vi "RSToutput.vi"(6 "RST Motor Constants":T1={"Pitch Gain (2*pi/enc)"=1.0, "Output Sign"=[1.0, -1.0, 1.0], "Phase Offset (rad)"=0.0, "Saturation"=32000.0}, 9 "Encoder Position":dbl, 11 "Command":dbl) -> (1 "Coerced?":bool, 3 "Control":dbl[](array[numeric]))   [LabVIEW 2010, in "kevLib2010.lvlib"]
uses:
  kevLib2010.lvlib
  RSTtypeDef.ctl
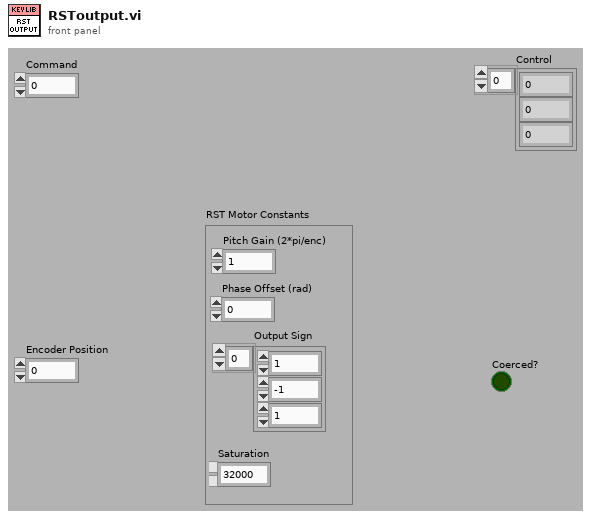
[diagram p1: front panel]
types:
  T1 = typedef "kevLib2010.lvlib/RSTtypeDef.ctl" = cluster{"Pitch Gain (2*pi/enc)":dbl, "Output Sign":dbl[], "Phase Offset (rad)":dbl, "Saturation":dbl}
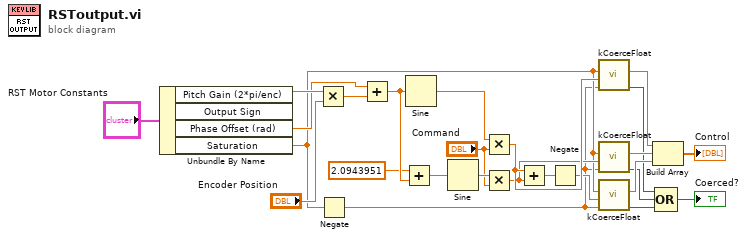
[diagram p0: block diagram]
diagram:
  n1 = Unbundle By Name("RST Motor Constants") -> ("Pitch Gain (2*pi/enc)"=w23:dbl, "Phase Offset (rad)"=w21:dbl, "Saturation"=w5:dbl)  [unwired: 1 out]
  n2 = Multiply(x=w23, y="Encoder Position") -> (x*y=w22:dbl)
  n3 = Negate(x=w5) -> (-x=w4:dbl)
  n4 = Add(x=w21, y=w22) -> (x+y=w3:dbl)
  n5 = Add(x=2.0943951, y=w3) -> (x+y=w2:dbl)
  n6 = Sine(x=w3) -> (sin(x)=w20:dbl)
  n7 = Sine(x=w2) -> (sin(x)=w19:dbl)
  n8 = Multiply(x=w20, y="Command") -> (x*y=w16:dbl)
  n9 = Multiply(x=w19, y="Command") -> (x*y=w14:dbl)
  n10 = Add(x=w16, y=w14) -> (x+y=w17:dbl)
  n11 = Negate(x=w17) -> (-x=w15:dbl)
  n12 = call "kCoerceFloat.vi"("lower"=w4, "input"=w16, "upper"=w5) -> ("coerced?"=w10:bool, "output"=w13:dbl)  [unwired: 7 in]
  n13 = call "kCoerceFloat.vi"("lower"=w4, "input"=w14, "upper"=w5) -> ("coerced?"=w9:bool, "output"=w12:dbl)  [unwired: 7 in]
  n14 = call "kCoerceFloat.vi"("lower"=w4, "input"=w15, "upper"=w5) -> ("coerced?"=w8:bool, "output"=w11:dbl)  [unwired: 7 in]
  n15 = Build Array(w13, w12, w11) -> (→"Control":dbl[])
  n16 = Compound Arithmetic op=OR(w10, w9, w8) -> (→"Coerced?":bool)
